vi "N6(problem).vi"() -> ()   [LabVIEW 2020]
uses:
  7f9115e3-b111-487f-af19-15bf33eaf760.vi
panel:
  out "spreadsheet string":string
  out "error out":errorcluster
  in  "file path (use dialog)":path
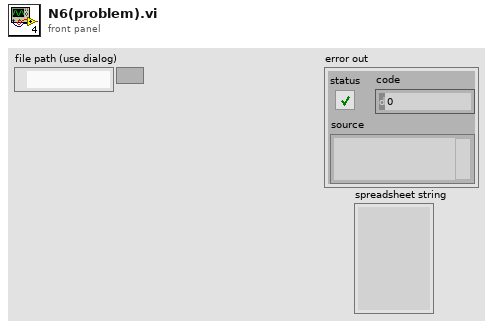
[diagram p1: front panel]
types:
  T1 = enum16{"open", "replace", "create", "open or create", "replace or create", "replace or create with confirmation"}
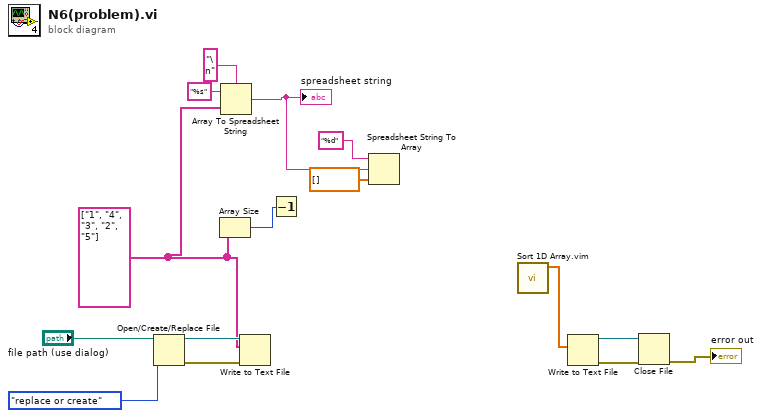
[diagram p0: block diagram]
diagram:
  w6 = string[] ["1", "4", "3", "2", "5"]
  n1 = Open/Create/Replace File(file path (use dialog)="file path (use dialog)", operation (0:open)=T1."replace or create") -> (refnum out=w14:refnum<file>, error out=w13:errorcluster)  [unwired: 4 in, 1 out]
  n2 = Array Size(array=w6) -> (size(s)=w7:i32)
  n3 = Array To Spreadsheet String(delimiter (Tab)="\n", array=w6, 3:"%s" ("format string")) -> (spreadsheet string=w3:string)
  "spreadsheet string" <- w3
  n4 = Write to Text File(file (use dialog)=w14, text=w6, error in=w13) -> ()  [unwired: 1 in, 3 out]
  n5 = Decrement(x=w7) -> ()  [unwired: 1 out]
  n6 = Spreadsheet String To Array(format string="%d", spreadsheet string=w3, array type (2D Dbl)=dbl[] []) -> ()  [unwired: 1 in, 1 out]
  n7 = call "Sort 1D Array.vim"() -> ("sorted array"=w11:dbl[])  [unwired: 11 in]
  n8 = Write to Text File(text=w11) -> (refnum out=w10:refnum<file>, error out=w9:errorcluster)  [unwired: 3 in, 1 out]
  n9 = Close File(refnum=w10, error in=w9) -> (error out=→"error out":errorcluster)  [unwired: 1 out]
